vi "baseline_c_with_timing.vi"() -> ()   [LabVIEW 2013]
uses:
  project/Baseline/Release/Baseline.dll
panel:
  out "time (ms)":dbl format="%#_13g"
  out "baseline":dbl format="%#_13g"
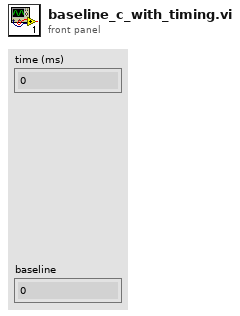
[diagram p1: front panel]
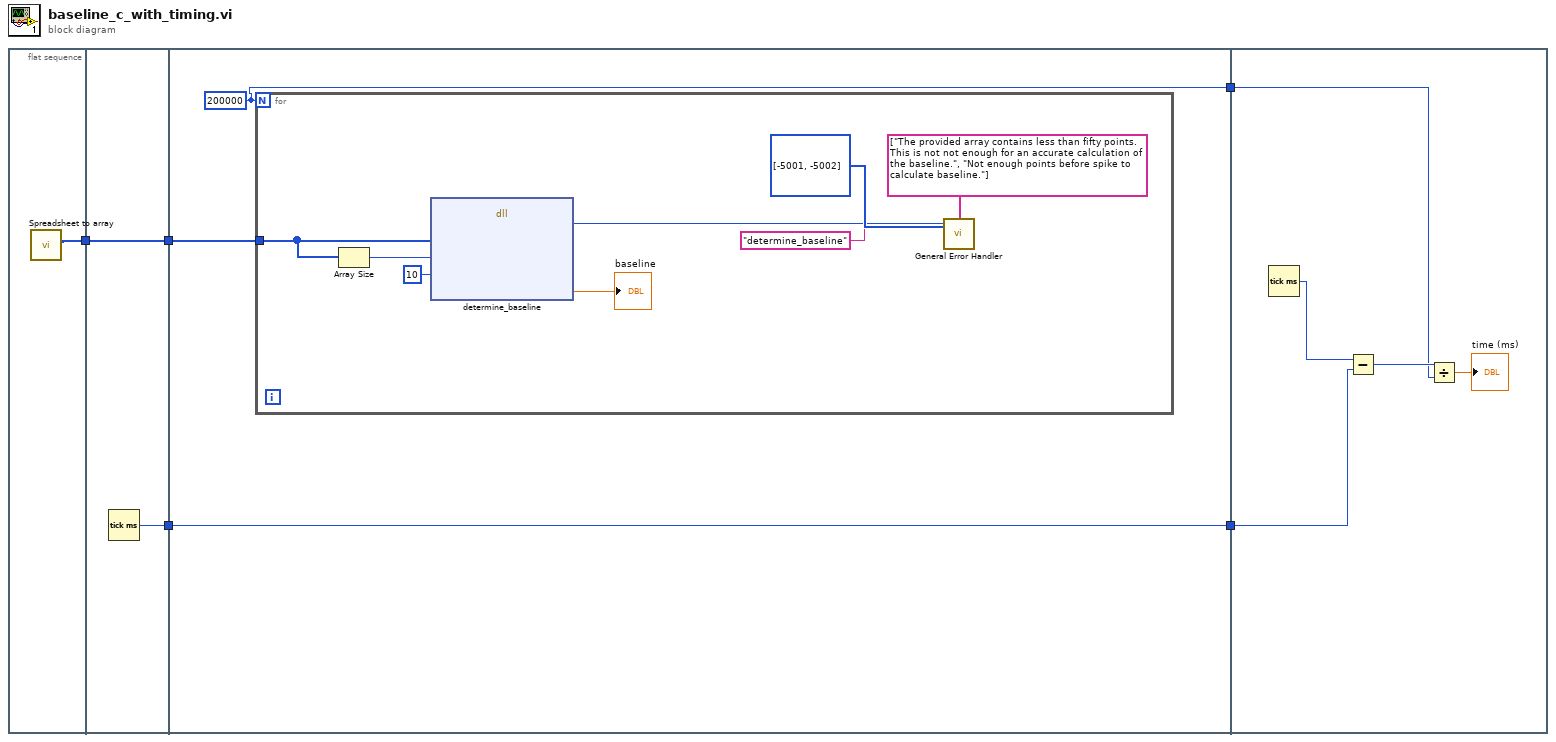
[diagram p0: block diagram]
diagram:
  n1 = flat-sequence {
    tunnel: [w6] -> w5
    tunnel: w5 -> [w8]
    tunnel: [w8] -> w4
    tunnel: [w7] -> w3
    tunnel: w4 -> [w11]
    tunnel: w3 -> [w10]
    tunnel: [w10] -> w2
    tunnel: [w9] -> w1
    tunnel: w2 -> [w23]
    tunnel: w1 -> [w21]
    frame #0 {
      n2 = call "Spreadsheet to array.vi"() -> ("Array"=w6:u16[])  [unwired: 8 in, 3 out]
    }
    frame #1 {
      n3 = Tick Count (ms)() -> (millisecond timer value=w7:u32)
    }
    frame #2 {
      w9 = 200000
      n4 = for {
        N: w9 -> [_]
        tunnel: w11 -> [w12]
        n5 = Array Size(array=w12) -> (size(s)=w19:i32)
        n6 = dll-call lib="C:/Users/SuperUser/Documents/HiSparc/Filter/C/project/Baseline/Release/Baseline.dll" fn="determine_baseline"("adValues"=w12, "size"=w19, "threshold"=10) -> ("error"=w14:i32, "baseline"=→"baseline":dbl)  [unwired: 7 in, 2 out]
        n7 = call <vilib>:"General Error Handler.vi"("[error code] (0)"=w14, "[user-defined codes]"=i32[] [-5001, -5002], "[user-defined descriptions]"=string[] ["The provided array contains less than fifty points. This is not not enough for an accurate calculation of the baseline.", "Not enough points before spike to calculate baseline."], "[error source] (\" \")"="determine_baseline" ("[error source] (\" \")")) -> ()  [unwired: 7 in, 5 out]
      }
    }
    frame #3 {
      n8 = Tick Count (ms)() -> (millisecond timer value=w24:u32)
      n9 = Subtract(x=w24, y=w23) -> (x-y=w22:u32)
      n10 = Divide(x=w22, y=w21) -> (x/y=→"time (ms)":dbl)
    }
  }
